vi "example 1 - plot.vi"() -> ()   [LabVIEW 2020]
uses:
  ui-testing/ui-testing.lvlib
panel:
  out "Plot":dbl[](graph)
  in  "Random":bool
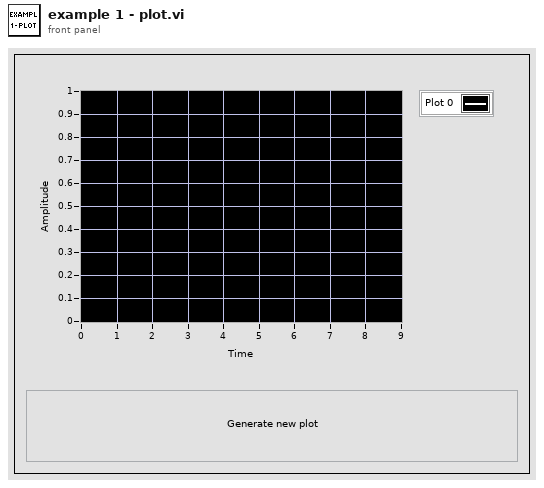
[diagram p1: front panel]
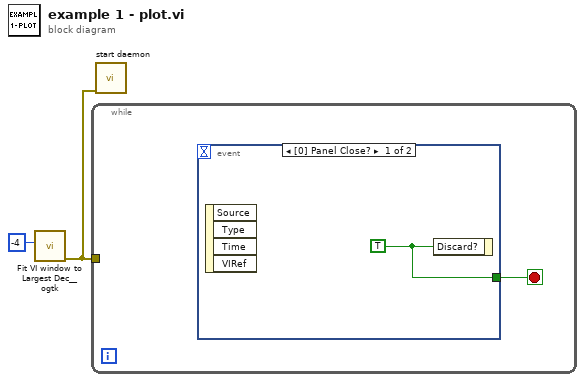
[diagram p0: block diagram]
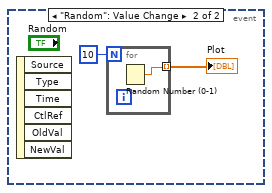
[diagram p2: hidden frame]
diagram:
  n1 = call <userlib>:"Fit VI window to Largest Dec__ogtk.vi"("border spacing (2 px)"=-4) -> ("error out"=w1:errorcluster)  [unwired: 5 in, 1 out]
  n2 = while {
    tunnel: w1 -> [_]
    stop <- w3 stop-if-true
    n3 = event shown="[0] Panel Close?" {
      selector: _ -> [_ _]
      dyn-events: _ -> [_ _]
      timeout: _ -> [_ _]
      tunnel: [w4 _] -> w3
      event Panel Close? {
        w4 = TRUE
        n4 = event-data() -> ()  [unwired: 1 in, 4 out]
        n5 = event-data("Discard?"=w4) -> ()  [unwired: 1 in, 1 out]
      }
      event "Random": Value Change {
        n6 = event-data() -> ()  [unwired: 1 in, 6 out]
        n7 = for {
          N: 10 -> [_]
          tunnel: [w7] -> w5 mode=indexing
          n8 = Random Number (0-1)() -> (number: 0 to 1=w7:dbl)
        }
        "Plot" <- w5
      }
    }
  }
  n9 = call "start daemon.vi"("error in (no error)"=w1) -> ()  [unwired: 10 in, 1 out]
